vi "Window-Enter new laser wavelength.vi"(8 "error in (no error)":errorcluster) -> (0 "error out":errorcluster, 1 "Cancelled":bool, 3 "Laser wavelength (nm)":u16 min=1 max=1 step=1)   [LabVIEW 2017]
doc: "Use this template to create a dialog box with event handling."
uses:
  <vilib>/Utility/miscctls.llb/LVPointTypeDef.ctl
  Global Variables/General Globals.vi
panel:
  in  "Cancel":bool
  in  "Laser wavelength":u16 max=10000 step=1 format="%.0f nm"
  in  "OK":bool
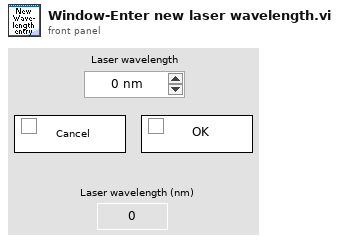
[diagram p1: front panel]
types:
  T1 = typedef "LVPointTypeDef.ctl" = cluster{"Horizontal":i16, "Vertical":i16}
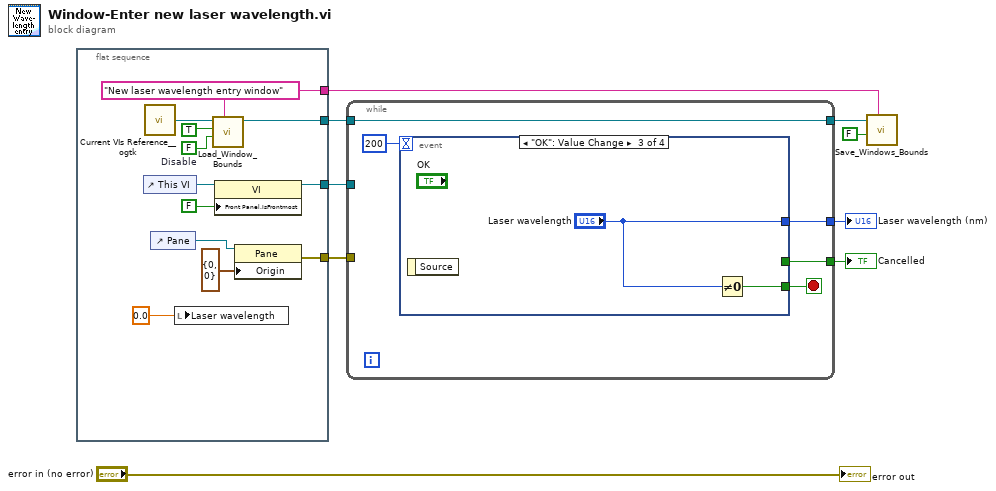
[diagram p0: block diagram]
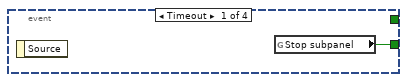
[diagram p2: hidden frame]
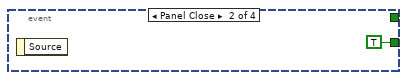
[diagram p3: hidden frame]
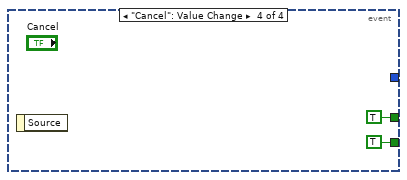
[diagram p4: hidden frame]
diagram:
  n1 = flat-sequence {
    tunnel: [w19] -> w9
    tunnel: [w17] -> w8
    tunnel: [w13] -> w7
    tunnel: [w12] -> w6
    frame #0 {
      w14 = FALSE  # Disable
      w13 = "New laser wavelength entry window" ("Window Name (i.e. Key)")
      n2 = control-ref of="This VI"() -> (w20:refnum<vi>)
      n3 = call <userlib>:"Current VIs Reference__ogtk.vi"() -> ("Current VI's reference"=w15:refnum<vi>)  [unwired: 5 in]
      n4 = control-ref of="Pane"() -> (w16:refnum<vi>)
      n5 = local write "Laser wavelength"(0.0 ("Requested trigger pulse width (ms)")) -> ()
      n6 = call "Load_Window_Bounds.vi"("Window Name (i.e. Key)"=w13, "Disable"=w14, "First Call"=TRUE, "Window VI's Ref"=w15) -> ("reference out"=w12:refnum<vi>)  [unwired: 4 in, 3 out]
      n7 = property on="Property Node" class="VI"(reference=w20, "Front Panel.IsFrontmost"=FALSE ("Front Panel Window:Is Frontmost")) -> (reference out=w19:refnum<vi>)  [unwired: 1 in, 1 out]
      n8 = property class="Pane"(reference=w16, "Origin"=T1 {"Horizontal"=0, "Vertical"=0}) -> (error out=w17:errorcluster)  [unwired: 1 in, 1 out]
    }
  }
  n9 = while {
    tunnel: w8 -> [_]
    tunnel: w9 -> [_]
    tunnel: w6 -> [w24]
    tunnel: [w24] -> w5
    tunnel: [w23] -> w2
    tunnel: [w22] -> w1
    stop <- w26 stop-if-true
    n10 = event shown="[2] \"OK\": Value Change" {
      selector: _ -> [_ _ _ _]
      dyn-events: _ -> [_ _ _ _]
      timeout: 200 -> [_ _ _ _]
      tunnel: [w27 TRUE ("Stop?") w29 TRUE ("Stop?")] -> w26
      tunnel: [_ _ _ TRUE ("Stop?")] -> w23
      tunnel: [_ _ "Laser wavelength" _] -> w22
      event Timeout {
        n11 = event-data() -> ()  [unwired: 1 in, 1 out]
        n12 = global read "General Globals.vi" "Stop subpanel"() -> (w27:bool)
      }
      event Panel Close {
        n13 = event-data() -> ()  [unwired: 1 in, 1 out]
      }
      event "OK": Value Change {
        n14 = event-data() -> ()  [unwired: 1 in, 1 out]
        n15 = Not Equal To 0?(x="Laser wavelength") -> (x != 0?=w29:bool)
      }
      event "Cancel": Value Change {
        n16 = event-data() -> ()  [unwired: 1 in, 1 out]
      }
    }
  }
  "Cancelled" <- w2
  "Laser wavelength (nm)" <- w1
  n17 = call "Save_Windows_Bounds.vi"("Window Name (i.e. Key)"=w7, "Front Panel Window:Open"=FALSE, "Window VI's Ref"=w5) -> ()  [unwired: 8 in, 1 out]
  "error out" <- "error in (no error)"
